vi "Set Field North.vi"(8 "error in (no error)":errorcluster, 11 "Turret in":refnum<class "Turret.lvclass">) -> (0 "error out":errorcluster, 3 "Turret out":refnum<class "Turret.lvclass">)   [LabVIEW 2019, in "Turret.lvlib" / "Turret.lvclass"]
uses:
  Turret.lvclass
  <vilib>/Rock Robotics/WPI/ThirdParty/Phoenix-LabVIEW/Pigeon IMU/CTRE_PigeonIMU_TareType.ctl
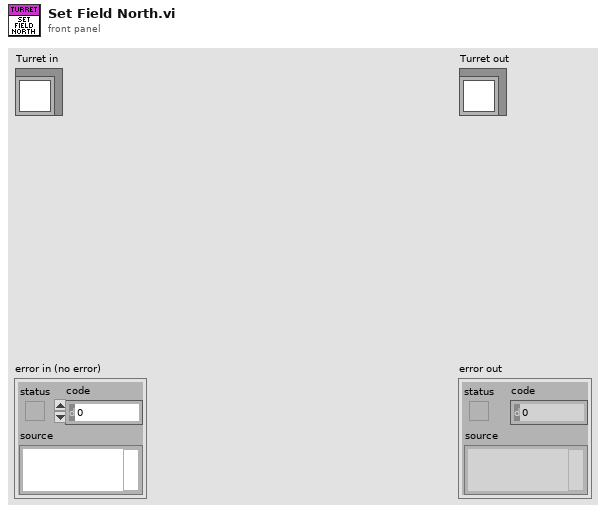
[diagram p1: front panel]
types:
  T1 = typedef "CTRE_PigeonIMU_TareType.ctl" = u8
  T2 = typedef "CTRE_PigeonIMU_DeviceRef.ctl" = cluster{"DeviceStatus":errorcluster, "Device Number":u8, "Type":T3, "Device ID":u32, "Handle":u64, "UsageFrame":u32, "Library Path":path}
  T3 = typedef "CTRE_PigeonIMU_ConnectionType.ctl" = u32
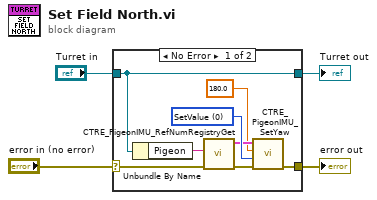
[diagram p0: block diagram]
diagram:
  n1 = case shown="No Error" "error in (no error)" {
    selector: "error in (no error)" -> [w8 w14]
    tunnel: [w7 w14] -> w3
    tunnel: [w12 w13] -> w1
    tunnel: "Turret in" -> [w12 w13]
    frame No Error {
      w11 = T1 0 items=["SetValue"=0, "AddOffset"=1, "MatchCompass"=2, "SetOffset"=255] ("TareType (SetValue)")
      n2 = Unbundle By Name(w12) -> ("Pigeon"=w5:string)
      n3 = call <vilib>:"CTRE_PigeonIMU_RefNumRegistryGet.vi"("error in (no error)"=w8, "refnum name"=w5) -> ("error out"=w9:errorcluster, "PigeonIMUDevRef"=w10:T2)  [unwired: 8 in]
      n4 = call <vilib>:"CTRE_PigeonIMU_SetYaw.vi"("error in (no error)"=w9, "TareType (SetValue)"=w11, "Value"=180.0, "PigeonIMUDevRef"=w10) -> ("error out"=w7:errorcluster)  [unwired: 6 in, 1 out]
    }
    frame Error {
    }
  }
  "error out" <- w3
  "Turret out" <- w1
